vi "Day 17 Puzzle 1.vi"(11 "Path":path) -> ()   [LabVIEW 2021]
uses:
  <vilib>/Utility/file.llb/Read Delimited Spreadsheet (string).vi
panel:
  out "size(s)":i32[](array[numeric])
  out "Current layout":string[][](array[string])
  out "rows":i32
  out "Array":string[](array[string])
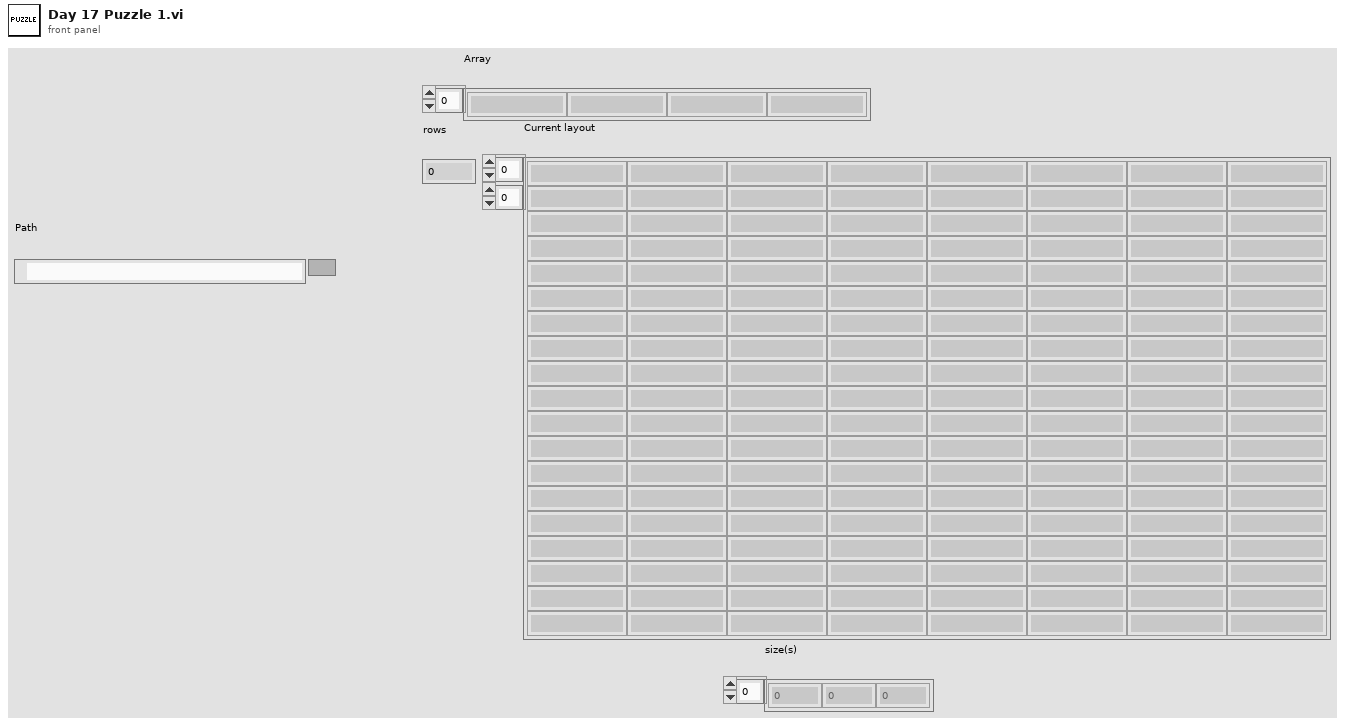
[diagram p1: front panel]
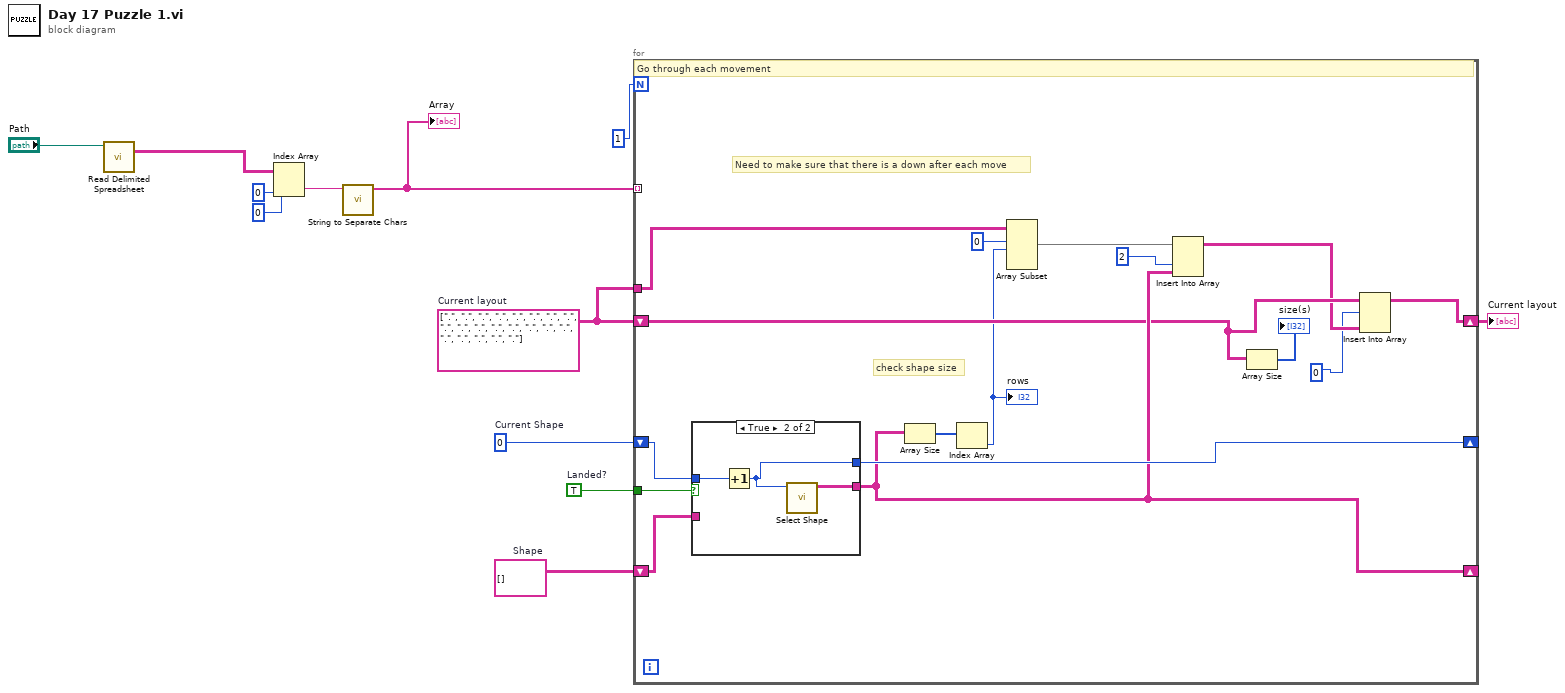
[diagram p0: block diagram]
diagram:
  w3 = string[][] []  # Shape
  w4 = TRUE  # Landed?
  w6 = 0  # Current Shape
  w5 = string[][] [[".", ".", ".", ".", ".", ".", "."], [".", ".", ".", ".", ".", ".", "."], [".", ".", ".", ".", ".", ".", "."]]  # Current layout
  n1 = call-poly <vilib>:"Read Delimited Spreadsheet.vi"("file path (dialog if empty)"="Path") -> ("all rows"=w11:string[][])  [unwired: 9 in, 5 out]
  n2 = Index Array(array=w11, index (row)=0 ("disabled index (row)"), index (col)=0 ("disabled index (col)")) -> (element=w8:string)
  n3 = call "String to Separate Chars.vi"("String"=w8) -> ("Array"=w7:string[])  [unwired: 10 in]
  "Array" <- w7
  n4 = for {
    N: 1 -> [_]
    shift-right: [w15] -> w1
    shift-left: w5 -> [w22]
    tunnel: w7 -> [_] mode=indexing
    shift-right: [w25] -> _
    shift-left: w6 -> [w27]
    tunnel: w5 -> [w16]
    tunnel: w4 -> [w28]
    shift-right: [w23] -> _
    shift-left: w3 -> [w26]
    # "check shape size"
    # "Need to make sure that there is a down after each move"
    # "Go through each movement"
    n5 = case shown="True" w28 {
      tunnel: w27 -> [w29 w32]
      tunnel: [w30 w33] -> w23
      tunnel: w26 -> [w30 _]
      tunnel: [w29 w31] -> w25
      frame False {
      }
      frame True {
        n6 = Increment(x=w32) -> (x+1=w31:i32)
        n7 = call "Select Shape.vi"("Numeric"=w31) -> ("Shape"=w33:string[][])  [unwired: 10 in]
      }
    }
    n8 = Array Size(array=w23) -> (size(s)=w24:i32[])
    n9 = Index Array(array=w24) -> (element=w19:i32)  [unwired: 1 in]
    "rows" <- w19
    n10 = Array Subset(array=w16, index (row)=0 ("index"), length (row)=w19) -> (w18:string[][])  [unwired: 2 in]
    n11 = Insert Into Array(array=w18, index (col)=2 ("index (row)"), new element=w23) -> (w14:string[][])  [unwired: 1 in]
    n12 = Array Size(array=w22) -> (size(s)=→"size(s)":i32[])
    n13 = Insert Into Array(array=w22, index (row)=0, new element=w14) -> (w15:string[][])  [unwired: 1 in]
  }
  "Current layout" <- w1
